vi "Lower Case No Space String.vi"(1 "String":string) -> (0 "Lower Case No Space String":string)   [LabVIEW 2021, in "Strings.lvlib"]
doc: "Removes all invisible characters (including end of line, etc) and underscore characters.\n\nUse this VI to simplify comparison with a target pattern(s)."
uses:
  Strings.lvlib
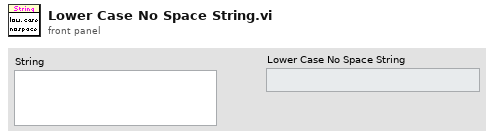
[diagram p1: front panel]
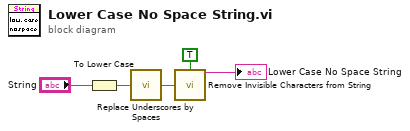
[diagram p0: block diagram]
diagram:
  n1 = To Lower Case(string="String") -> (all lower case string=w3:string)
  n2 = call "Replace Underscores by Spaces.vi"("String in"=w3) -> ("String out"=w1:string)  [unwired: 8 in]
  n3 = call "Remove Invisible Characters from String.vi"("Remove Line Feed. etc (F)"=TRUE, "String"=w1) -> ("result string"=→"Lower Case No Space String":string)  [unwired: 2 in]
